vi "Get Packet Type (1st Element).vi"(9 "1st Packet Element":u8) -> (0 "End":bool, 3 "Return Packet Type":T1)   [LabVIEW 2014, in "hse-db.lvlib" / "MySQL (TCP).lvlib"]
uses:
  MySQL (TCP).lvlib
  Controls/Return Packet Types.ctl
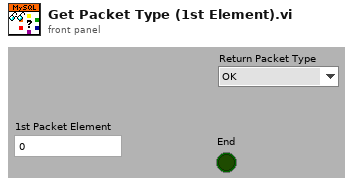
[diagram p1: front panel]
types:
  T1 = typedef "hse-db.lvlib/MySQL (TCP).lvlib/Return Packet Types.ctl" = enum16{"OK", "Result Set Header", "Error", "Field", "Row", "EOF"}
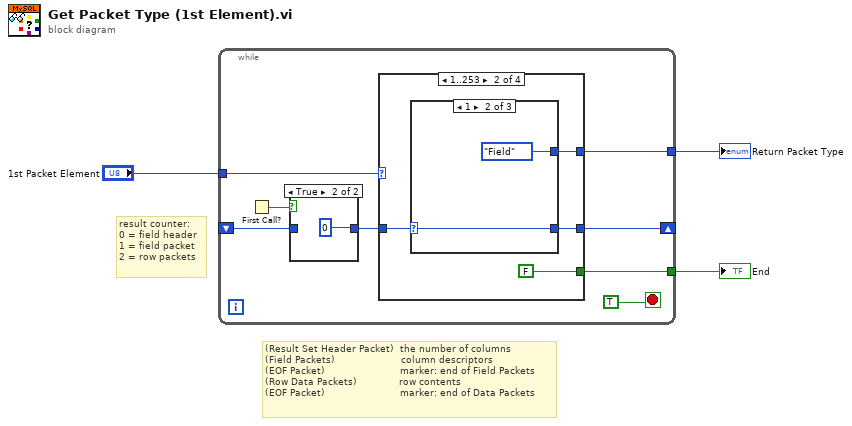
[diagram p0: block diagram]
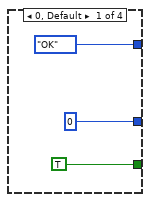
[diagram p3: hidden frame]
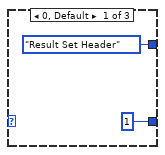
[diagram p4: hidden frame]
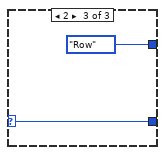
[diagram p5: hidden frame]
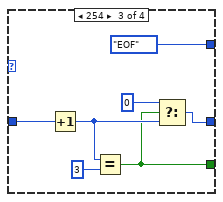
[diagram p6: hidden frame]
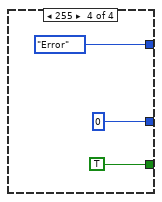
[diagram p7: hidden frame]
diagram:
  # "(Result Set Header Packet)  the number of columns\n(Field Packets)                      column descriptors\n(EOF Packet)                         marker: end of Field Packets\n(Row Data Packets)              row contents\n(EOF Packet)                         marker: end of Data Packets"
  # "result counter:\n0 = field header\n1 = field packet\n2 = row packets"
  n1 = while {
    tunnel: "1st Packet Element" -> [w11]
    tunnel: [w10] -> w2
    tunnel: [w9] -> w1
    shift-right: [w8] -> _
    shift-left: _ -> [w4]
    stop <- TRUE stop-if-true
    n2 = First Call?() -> (First Call?: T/F=w6:bool)
    n3 = case shown="True" w6 {
      tunnel: [w12 u8 0 ("Counter")] -> w5
      tunnel: w4 -> [w12 _]
      frame False {
      }
      frame True {
      }
    }
    n4 = case shown="1..253" w11 {
      tunnel: [Return_Packet_Types."OK" ("Previous Packet Type 2") w19 Return_Packet_Types."EOF" ("Previous Packet Type 2") Return_Packet_Types."Error" ("Previous Packet Type 2")] -> w10
      tunnel: w5 -> [_ w18 w31 _]
      tunnel: [u8 0 ("Counter") w17 w28 u8 0 ("Counter")] -> w8
      tunnel: [TRUE FALSE w27 TRUE] -> w9
      frame 0, Default {
      }
      frame 1..253 {
        n5 = case shown="1" w18 {
          selector: w18 -> [_ w23 w25]
          tunnel: [Return_Packet_Types."Result Set Header" ("Previous Packet Type 2") Return_Packet_Types."Field" ("Previous Packet Type 2") Return_Packet_Types."Row" ("Previous Packet Type 2")] -> w19
          tunnel: [u8 1 w23 w25] -> w17
          frame 0, Default {
          }
          frame 1 {
          }
          frame 2 {
          }
        }
      }
      frame 254 {
        n6 = Increment(x=w31) -> (x+1=w29:u8)
        n7 = Equal?(x=w29, y=u8 3) -> (x = y?=w27:bool)
        n8 = Select(t=u8 0, s=w27, f=w29) -> (s? t:f=w28:u8)
      }
      frame 255 {
      }
    }
  }
  "Return Packet Type" <- w2
  "End" <- w1
